vi "test_GetItemInfosFromProjectFile_EmptyProject.vi"() -> (3 "Pass?":bool)   [LabVIEW 2019, in "Tests.SolutionBuilder.lvlib"]
uses:
  Tests.SolutionBuilder.lvlib
  SolutionBuilder/SolutionBuilder.lvclass
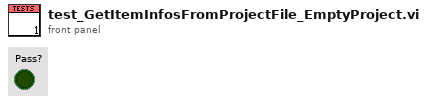
[diagram p1: front panel]
types:
  T1 = typedef "SolutionBuilder.lvlib/SolutionBuilder.lvclass/ProjectItemMap.ctl" = map{path, refnum<class "ProjectItem.lvclass">[]}
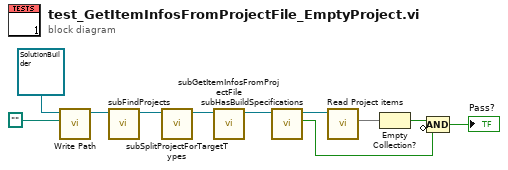
[diagram p0: block diagram]
diagram:
  n1 = call "Write Path.vi"("Path"=path "", "SolutionBuilder in"=refnum<class "SolutionBuilder.lvclass"> refnum) -> ("SolutionBuilder out"=w10:refnum<class "SolutionBuilder.lvclass">)  [unwired: 9 in]
  n2 = call "subFindProjects.vi"("SolutionBuilder in"=w10) -> ("SolutionBuilder out"=w2:refnum<class "SolutionBuilder.lvclass">)  [unwired: 9 in, 1 out]
  n3 = call "subSplitProjectForTargetTypes.vi"("SolutionBuilder in"=w2) -> ("SolutionBuilder out"=w1:refnum<class "SolutionBuilder.lvclass">)  [unwired: 9 in, 1 out]
  n4 = call "subGetItemInfosFromProjectFile.vi"("SolutionBuilder in"=w1) -> ("SolutionBuilder out"=w6:refnum<class "SolutionBuilder.lvclass">)  [unwired: 9 in, 1 out]
  n5 = call "subHasBuildSpecifications.vi"("SolutionBuilder in"=w6) -> ("Has specs?"=w4:bool, "SolutionBuilder out"=w5:refnum<class "SolutionBuilder.lvclass">)  [unwired: 8 in, 1 out]
  n6 = call "Read Project items.vi"("SolutionBuilder in"=w5) -> ("Project items"=w8:T1)  [unwired: 9 in, 1 out]
  n7 = Empty Collection?(1:w8) -> (0:w7:bool)
  n8 = Compound Arithmetic op=AND(w7, invert w4) -> (→"Pass?":bool)
